vi "Drive_Utils_RealCoG.vi"(8 "error in (no error)":errorcluster, 9 "Y relative":dbl, 10 "X relative":dbl) -> (0 "error out":errorcluster, 1 "Angle b":dbl, 2 "Radius r":dbl)   [LabVIEW 2009, in "Drive.lvlib" / "Drive_Utils.lvlib"]
uses:
  Drive_Utils.lvlib
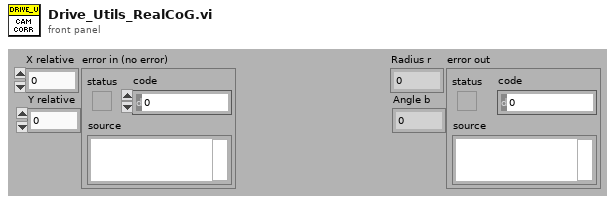
[diagram p1: front panel]
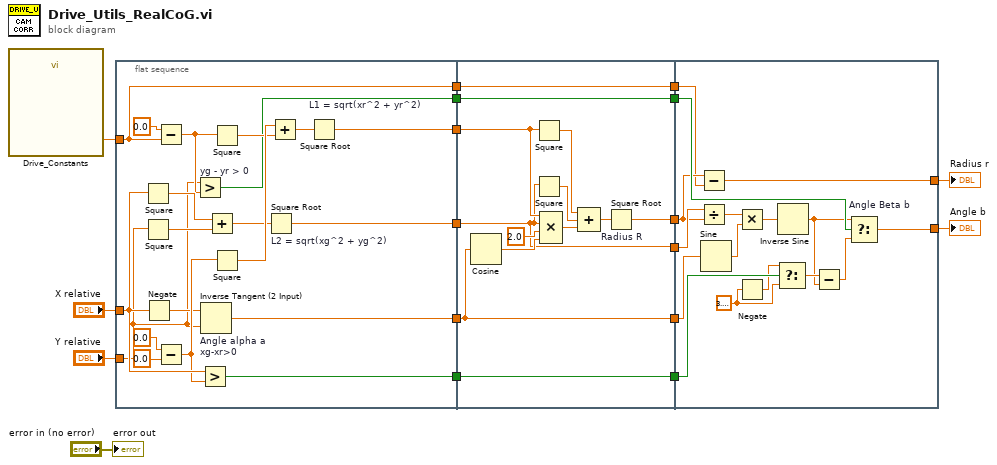
[diagram p0: block diagram]
diagram:
  n1 = call "Drive_Constants.vi"() -> ("Camera Offset"=w2:dbl)  [unwired: 19 in, 8 out]
  n2 = flat-sequence {
    tunnel: "Y relative" -> [w19]
    tunnel: "X relative" -> [w27]
    tunnel: [w30] -> w16
    tunnel: [w29] -> w15
    tunnel: [w28] -> w14
    tunnel: [w23] -> w11
    tunnel: [w22] -> w9
    tunnel: w2 -> [w20]
    tunnel: [w20] -> w3
    tunnel: w16 -> [w40]
    tunnel: w15 -> [w41]
    tunnel: w14 -> [w51]
    tunnel: [w44] -> w13
    tunnel: [w43] -> w12
    tunnel: w11 -> [w43]
    tunnel: [w42] -> w10
    tunnel: w9 -> [w42]
    tunnel: [w41] -> w8
    tunnel: [w40] -> w7
    tunnel: [w39] -> w4
    tunnel: w3 -> [w39]
    tunnel: [w52] -> w6
    tunnel: w13 -> [w54]
    tunnel: w12 -> [w67]
    tunnel: w10 -> [w58]
    tunnel: w8 -> [w64]
    tunnel: w7 -> [w63]
    tunnel: [w57] -> w5
    tunnel: w4 -> [w53]
    frame #0 {
      n3 = Square(x=w27) -> (x^2=w31:dbl)
      n4 = Square(x=w19) -> (x^2=w25:dbl)
      n5 = Negate(x=w27) -> (-x=w21:dbl)
      n6 = Subtract(x=0.0, y=w20) -> (x-y=w24:dbl)
      n7 = Subtract(x=0.0, y=0.0) -> (x-y=w26:dbl)
      n8 = Greater? "yg - yr > 0"(x=w19, y=w24) -> (0:w22:bool)
      n9 = Greater? "xg-xr>0"(x=w27, y=w26) -> (0:w23:bool)
      n10 = Inverse Tangent (2 Input) "Angle alpha a"(1:w19, 2:w21) -> (0:w30:dbl)
      n11 = Add(x=w31, y=w25) -> (x+y=w32:dbl)
      n12 = Square(x=w24) -> (x^2=w36:dbl)
      n13 = Square(x=w26) -> (x^2=w37:dbl)
      n14 = Square Root "L2 = sqrt(xg^2 + yg^2)"(x=w32) -> (sqrt(x)=w29:dbl)
      n15 = Add(x=w37, y=w36) -> (x+y=w38:dbl)
      n16 = Square Root "L1 = sqrt(xr^2 + yr^2)"(x=w38) -> (sqrt(x)=w28:dbl)
    }
    frame #1 {
      n17 = Cosine(x=w40) -> (cos(x)=w49:dbl)
      n18 = Square(x=w51) -> (x^2=w46:dbl)
      n19 = Square(x=w41) -> (x^2=w47:dbl)
      n20 = Compound Arithmetic op=MULTIPLY(w51, w41, 2.0 ("value"), w49) -> (w48:dbl)
      n21 = Compound Arithmetic op=ADD(w46, w47, w48) -> (w45:dbl)
      n22 = Square Root "Radius R"(x=w45) -> (sqrt(x)=w44:dbl)
    }
    frame #2 {
      w65 = 3.141592653589793
      n23 = Subtract(x=w54, y=w53) -> (x-y=w52:dbl)
      n24 = Divide(x=w64, y=w54) -> (x/y=w61:dbl)
      n25 = Sine(x=w63) -> (sin(x)=w62:dbl)
      n26 = Multiply(x=w61, y=w62) -> (x*y=w56:dbl)
      n27 = Negate(x=w65) -> (-x=w66:dbl)
      n28 = Select(t=w66, s=w67, f=w65) -> (s? t:f=w60:dbl)
      n29 = Inverse Sine(1:w56) -> (0:w55:dbl)
      n30 = Subtract(x=w60, y=w55) -> (x-y=w59:dbl)
      n31 = Select "Angle Beta b"(t=w55, s=w58, f=w59) -> (s? t:f=w57:dbl)
    }
  }
  "Radius r" <- w6
  "Angle b" <- w5
  "error out" <- "error in (no error)"
